vi "Configure Hardware.vi"(8 "error in (no error)":errorcluster, 11 "Hardware Resources in":T2={"VISA resource name"="", "DAQ Type"=0, "Channel 1"={"Acquiring"=FALSE, "Enabled"=FALSE, "Terminal configuration"=32767, "Range"=0, "Coupling"=0}, "Channel 2"={"Acquiring"=FALSE, "Enabled"=FALSE, "Terminal configuration"=0, "Range"=0, "Coupling"=0}, "Timing"={"Sample Time [Time Units]"=0, "Actual Sample Time [s]"=0.0, "Samples per Iteration"=0, "Sample Clock Source"=0, "Time Units"=0, "t0"=timestamp(0 s since 1904-01-01), "Baud rate"=0}, "PS Parameters"={"PS handle"=0, "PS Max_adc"=32767, "PS Enabled Array"=[], "PS Device Info"={"Driver Version"="", "USB Version"="", "Hardware"="", "Variant"="", "Batch and Serial"="", "Cal Date"="", "Kernel Version"="", "Digital HW Version"="", "Analogue HW Version"="", "Firmware 1"="", "Firmware 2"="", "MSO"=FALSE, "Number of Channels"=0}, "Channel 1 Buffer"=refnum, "Channel 2 Buffer"=refnum, "Resolution"=0, "USB Power"=FALSE}, "Trigger"={"Direction"=0, "Threshold [V]"=0.0, "Enabled"=FALSE, "Trigger Source"=0}, "Keithley Parameters"={"Previous End / Current Start"=0, "Quantity"=0}} {"Keithley Parameters"."Quantity" items=["Current", "Voltage"]; "Trigger"."Trigger Source" items=["Channel 1"=0, "Channel 2"=1, "Ext."=4]; "Trigger"."Direction" items=["Falling", "Rising"]; "PS Parameters"."Resolution" items=["8", "12", "14", "15", "16"]; "Timing"."Time Units" items=["Seconds"]; "Timing"."Sample Clock Source" items=["Internal", "External"]; "Channel 2"."Coupling" items=["AC", "DC"]; "Channel 2"."Range" items=["0.01", "0.02", "0.05", "0.1", "0.2", "0.5", "1", "2", "5", "10", "20", "50", "100", "1000"]; "Channel 2"."Terminal configuration" items=["Referenced Single Ended", "Differential"]; "Channel 1"."Coupling" items=["AC", "DC"]; "Channel 1"."Range" items=["0.01", "0.02", "0.05", "0.1", "0.2", "0.5", "1", "2", "5", "10", "20", "50", "100", "1000"]; "Channel 1"."Terminal configuration" items=["Referenced Single Ended", "Differential"]; "DAQ Type" items=["Simulated", "Tektronics DPO2k/3k/4k", "PicoScope 2000a Series", "Keithley DMM7510", "PicoScope 5000a Series", "Arduino"]}) -> (0 "error out":errorcluster, 3 "Hardware Resources out":T2={"VISA resource name"="", "DAQ Type"=0, "Channel 1"={"Acquiring"=FALSE, "Enabled"=FALSE, "Terminal configuration"=32767, "Range"=0, "Coupling"=0}, "Channel 2"={"Acquiring"=FALSE, "Enabled"=FALSE, "Terminal configuration"=0, "Range"=0, "Coupling"=0}, "Timing"={"Sample Time [Time Units]"=0, "Actual Sample Time [s]"=0.0, "Samples per Iteration"=0, "Sample Clock Source"=0, "Time Units"=0, "t0"=timestamp(0 s since 1904-01-01), "Baud rate"=0}, "PS Parameters"={"PS handle"=0, "PS Max_adc"=32767, "PS Enabled Array"=[], "PS Device Info"={"Driver Version"="", "USB Version"="", "Hardware"="", "Variant"="", "Batch and Serial"="", "Cal Date"="", "Kernel Version"="", "Digital HW Version"="", "Analogue HW Version"="", "Firmware 1"="", "Firmware 2"="", "MSO"=FALSE, "Number of Channels"=0}, "Channel 1 Buffer"=refnum, "Channel 2 Buffer"=refnum, "Resolution"=0, "USB Power"=FALSE}, "Trigger"={"Direction"=0, "Threshold [V]"=0.0, "Enabled"=FALSE, "Trigger Source"=0}, "Keithley Parameters"={"Previous End / Current Start"=0, "Quantity"=0}} {"Keithley Parameters"."Quantity" items=["Current", "Voltage"]; "Trigger"."Trigger Source" items=["Channel 1"=0, "Channel 2"=1, "Ext."=4]; "Trigger"."Direction" items=["Falling", "Rising"]; "PS Parameters"."Resolution" items=["8", "12", "14", "15", "16"]; "Timing"."Time Units" items=["Seconds"]; "Timing"."Sample Clock Source" items=["Internal", "External"]; "Channel 2"."Coupling" items=["AC", "DC"]; "Channel 2"."Range" items=["0.01", "0.02", "0.05", "0.1", "0.2", "0.5", "1", "2", "5", "10", "20", "50", "100", "1000"]; "Channel 2"."Terminal configuration" items=["Referenced Single Ended", "Differential"]; "Channel 1"."Coupling" items=["AC", "DC"]; "Channel 1"."Range" items=["0.01", "0.02", "0.05", "0.1", "0.2", "0.5", "1", "2", "5", "10", "20", "50", "100", "1000"]; "Channel 1"."Terminal configuration" items=["Referenced Single Ended", "Differential"]; "DAQ Type" items=["Simulated", "Tektronics DPO2k/3k/4k", "PicoScope 2000a Series", "Keithley DMM7510", "PicoScope 5000a Series", "Arduino"]})   [LabVIEW 2017, in "Acquisition.lvlib"]
doc: "Configure the hardware."
uses:
  Acquisition.lvlib
  Hardware Configuration.ctl
  Signal Type.ctl
  Settings/Terminal Configuration.ctl
  Settings/Range.ctl
  Settings/Coupling.ctl
  Settings/Sampling Clock Source.ctl
  Settings/Time Units.ctl
  Settings/Resolution.ctl
  Settings/Trigger Direction.ctl
  Settings/Trigger Source.ctl
  Settings/Quantity.ctl
  support/DAQ Drivers/Tektronix DPO MSO 2000 4000 Series/Tektronix DPO MSO 2000 4000 Series.lvlib
  Settings/Settings.lvlib
panel:
  out "Range":T1 items=["10 u"=50, "100 u"=51, "1 m"=52, "10 m"=0, "20 m"=1, "50 m"=2, "100 m"=3, "200 m"=4, "500 m"=5, "1"=6, "2"=7, "3"=53, "5"=8, "10"=9, "20"=10, "50"=11, "100"=12, "700"=90, "1000"=13]
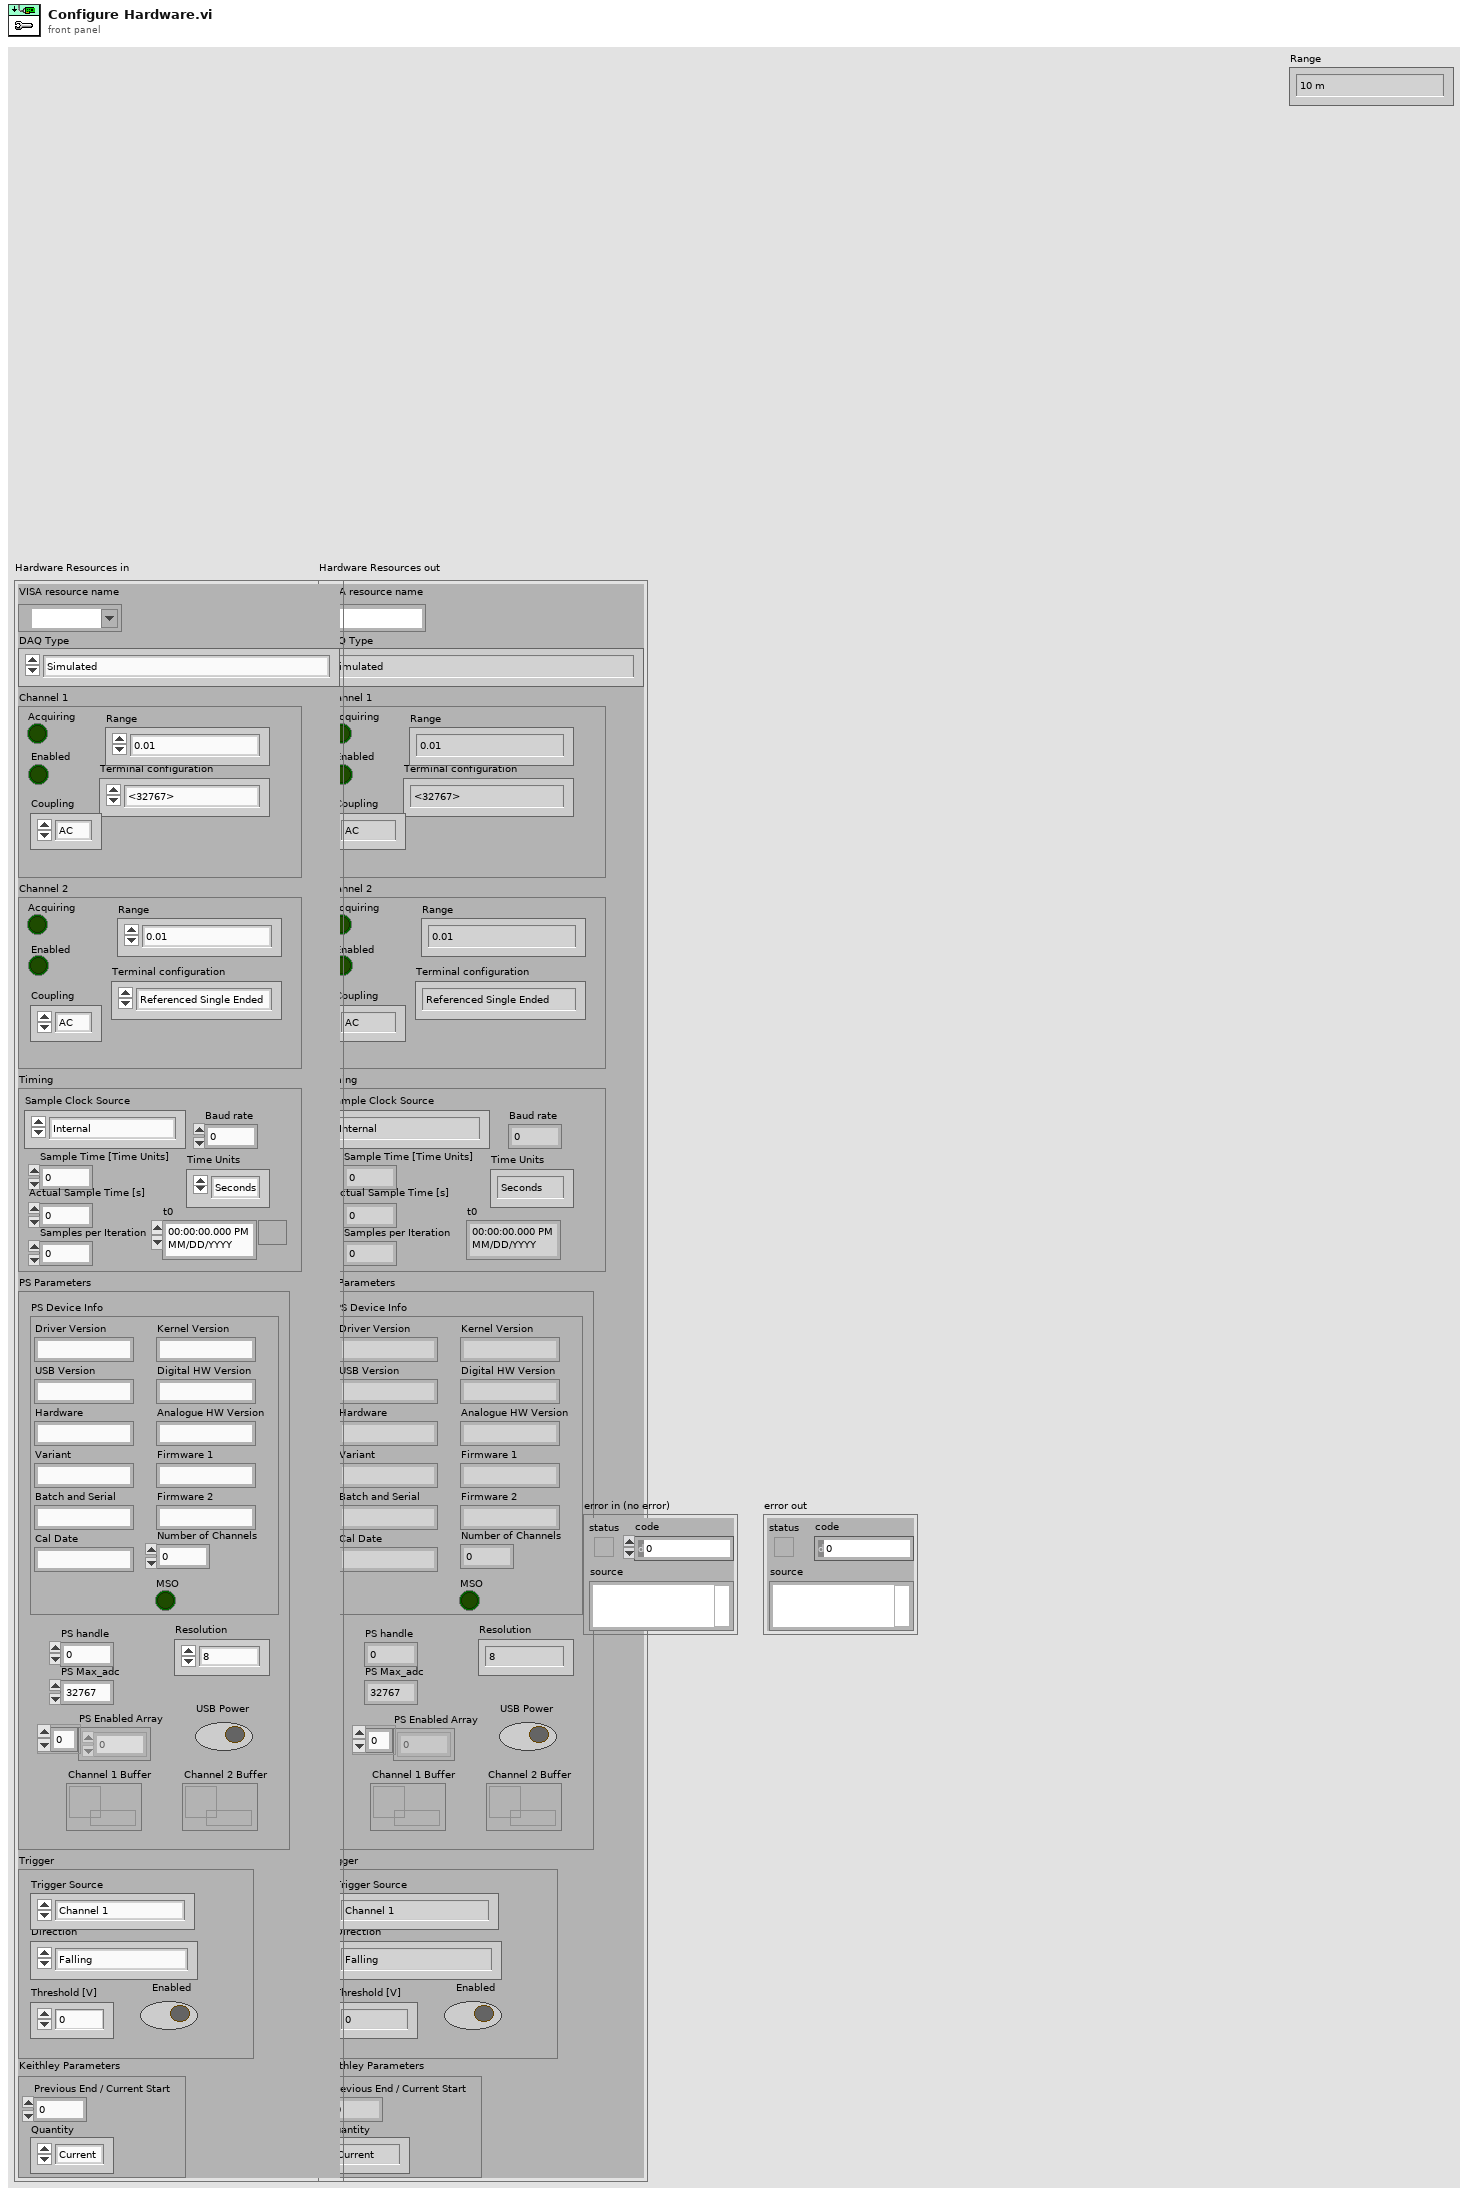
[diagram p1: front panel]
types:
  T1 = typedef "Settings.lvlib/Range.ctl" = u16
  T2 = typedef "Acquisition.lvlib/Hardware Configuration.ctl" = cluster{"VISA resource name":refnum<visa-resource-name>, "DAQ Type":T3, "Channel 1":cluster{"Acquiring":bool, "Enabled":bool, "Terminal configuration":T4, "Range":T1, "Coupling":T5}, "Channel 2":cluster{"Acquiring":bool, "Enabled":bool, "Terminal configuration":T4, "Range":T1, "Coupling":T5}, "Timing":cluster{"Sample Time [Time Units]":u32, "Actual Sample Time [s]":dbl, "Samples per Iteration":u32, "Sample Clock Source":T6, "Time Units":T7, "t0":timestamp, "Baud rate":u32}, "PS Parameters":cluster{"PS handle":i16, "PS Max_adc":i16, "PS Enabled Array":i16[], "PS Device Info":cluster{"Driver Version":string, "USB Version":string, "Hardware":string, "Variant":string, "Batch and Serial":string, "Cal Date":string, "Kernel Version":string, "Digital HW Version":string, "Analogue HW Version":string, "Firmware 1":string, "Firmware 2":string, "MSO":bool, "Number of Channels":i16}, "Channel 1 Buffer":refnum<data-value>, "Channel 2 Buffer":refnum<data-value>, "Resolution":T8, "USB Power":bool}, "Trigger":cluster{"Direction":T9, "Threshold [V]":dbl, "Enabled":bool, "Trigger Source":T10}, "Keithley Parameters":cluster{"Previous End / Current Start":i32, "Quantity":T11}}
  T3 = typedef "Acquisition.lvlib/Signal Type.ctl" = u16
  T4 = typedef "Settings.lvlib/Terminal Configuration.ctl" = u16
  T5 = typedef "Settings.lvlib/Coupling.ctl" = i16
  T6 = typedef "Settings.lvlib/Sampling Clock Source.ctl" = u16
  T7 = typedef "Settings.lvlib/Time Units.ctl" = u32
  T8 = typedef "Settings.lvlib/Resolution.ctl" = i32
  T9 = typedef "Settings.lvlib/Trigger Direction.ctl" = u16
  T10 = typedef "Settings.lvlib/Trigger Source.ctl" = u16
  T11 = typedef "Settings.lvlib/Quantity.ctl" = u16
  T12 = cluster{"Auto Stop":bool, "Desired Sample Interval":u32, "Pre-trigger Samples":u32, "Post-trigger Samples":u32, "Down-Sample Ratio":u32, "Down-Sample Mode":u32, "Overview Buffer Size":i32, "Time Units":u32}
  T13 = cluster{"Trigger Enabled":bool, "Trigger Source":enum16{"Channel A", "Channel B", "Channel C", "Channel D", "Ext."}, "Trigger Threshold (Volts)":dbl, "Trigger Direction":u16, "Trigger Delay (samples)":u32, "Auto Trigger Time (ms)":i16}
  T14 = cluster{"Auto Stop":bool, "Four Channel Device?":bool, "Desired Sample Interval":u32, "Pre-trigger Samples":u32, "Post-trigger Samples":u32, "Down-Sample Ratio":u32, "Down-Sample Mode":i32, "Overview Buffer Size":u32, "Time Units":u32}
  T15 = cluster{"Trigger Enabled":bool, "Trigger Source":enum16{"Channel A", "Channel B", "Channel C", "Channel D", "Ext."}, "Trigger Threshold (16-bit counts)":i16, "Trigger Direction":u16, "Trigger Delay (samples)":u32, "Auto Trigger Time (ms)":i16}
  T16 = cluster{"Acquiring":bool, "Enabled":bool, "Terminal configuration":T4, "Range":T1, "Coupling":T5}
  T17 = cluster{"Sample Time [Time Units]":u32, "Actual Sample Time [s]":dbl, "Samples per Iteration":u32, "Sample Clock Source":T6, "Time Units":T7, "t0":timestamp, "Baud rate":u32}
  T18 = cluster{"PS handle":i16, "PS Max_adc":i16, "PS Enabled Array":i16[], "PS Device Info":cluster{"Driver Version":string, "USB Version":string, "Hardware":string, "Variant":string, "Batch and Serial":string, "Cal Date":string, "Kernel Version":string, "Digital HW Version":string, "Analogue HW Version":string, "Firmware 1":string, "Firmware 2":string, "MSO":bool, "Number of Channels":i16}, "Channel 1 Buffer":refnum<data-value>, "Channel 2 Buffer":refnum<data-value>, "Resolution":T8, "USB Power":bool}
  T19 = cluster{"Direction":T9, "Threshold [V]":dbl, "Enabled":bool, "Trigger Source":T10}
  T20 = cluster{"Previous End / Current Start":i32, "Quantity":T11}
  T21 = cluster{"Enabled":bool, "Coupling":i16, "Range":u16, "Analogue Offset":sgl}
  T22 = cluster{"Driver Version":string, "USB Version":string, "Hardware":string, "Variant":string, "Batch and Serial":string, "Cal Date":string, "Kernel Version":string, "Digital HW Version":string, "Analogue HW Version":string, "Firmware 1":string, "Firmware 2":string, "MSO":bool, "Number of Channels":i16}
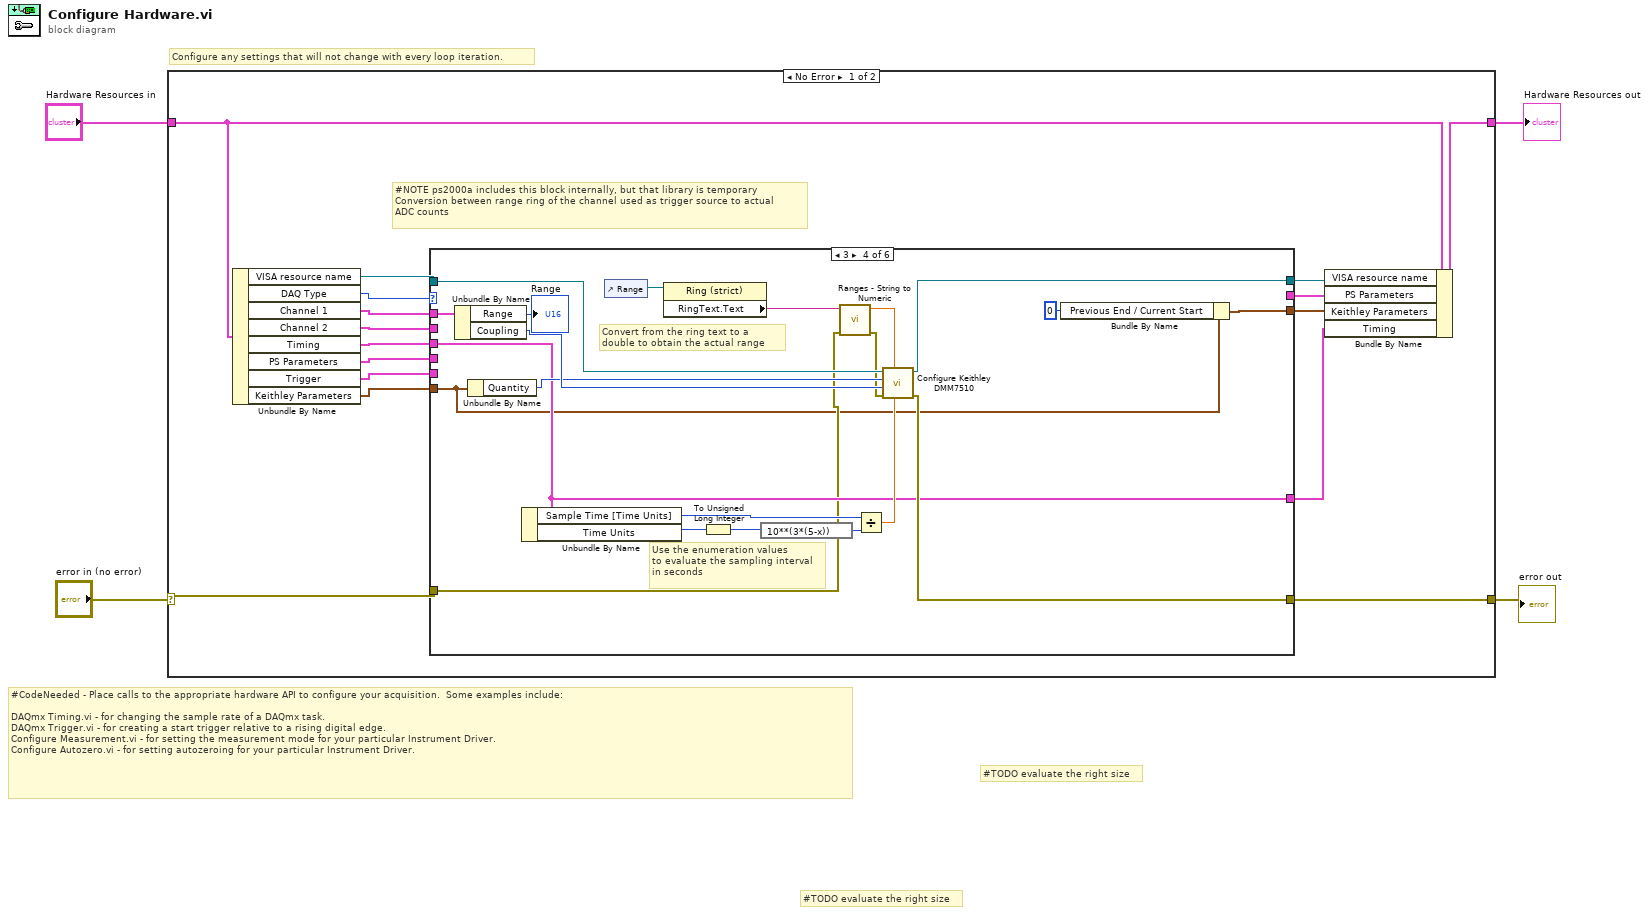
[diagram p0: block diagram]
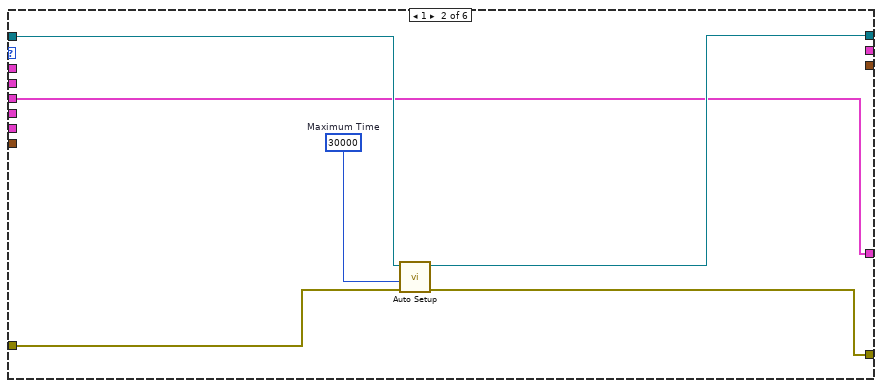
[diagram p3: hidden frame]
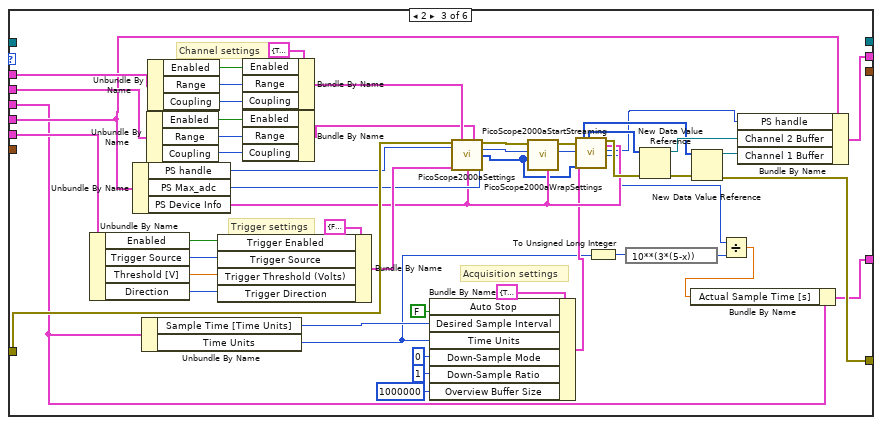
[diagram p4: hidden frame]
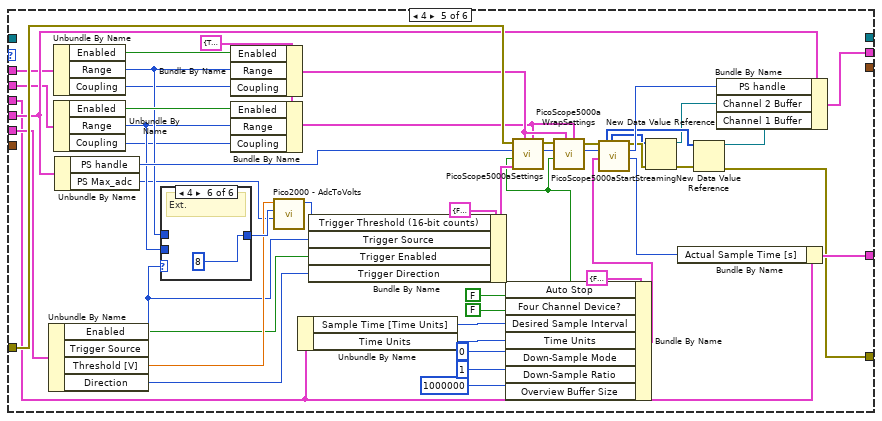
[diagram p5: hidden frame]
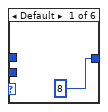
[diagram p6: hidden frame]
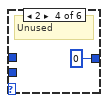
[diagram p9: hidden frame]
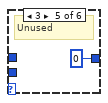
[diagram p10: hidden frame]
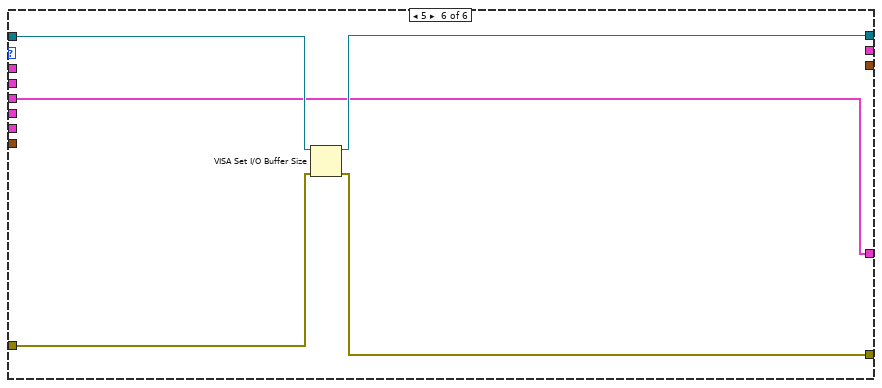
[diagram p11: hidden frame]
diagram:
  # "#TODO evaluate the right size"
  # "#TODO evaluate the right size"
  # "Configure any settings that will not change with every loop iteration."
  # "#CodeNeeded - Place calls to the appropriate hardware API to configure your acquisition.  Some examples include:\n\nDAQmx Timing.vi - for changing the sample rate of a DAQmx task.\nDAQmx Trigger.vi - for creating a start trigger relative to a rising digital edge.\nConfigure Measurement.vi - for setting the measurement mode for your particular Instrument Driver.\nConfigure Autozero.vi - for setting autozeroing for your particular Instrument Driver."
  n1 = case shown="No Error" "error in (no error)" {
    selector: "error in (no error)" -> [w19 w161]
    tunnel: [w18 w161] -> w3
    tunnel: "Hardware Resources in" -> [w16 w162]
    tunnel: [w20 w162] -> w1
    frame No Error {
      # "#NOTE ps2000a includes this block internally, but that library is temporary\nConversion between range ring of the channel used as trigger source to actual\nADC counts"
      n2 = Unbundle By Name(w16) -> ("VISA resource name"=w15:refnum<visa-resource-name>, "DAQ Type"=w14:T3, "Channel 1"=w13:T16, "Channel 2"=w11:T16, "Timing"=w12:T17, "PS Parameters"=w9:T18, "Trigger"=w10:T19, "Keithley Parameters"=w6:T20)
      n3 = case shown="3" w14 {
        tunnel: w19 -> [w22 w28 w77 w84 w149 w157]
        tunnel: [w22 w27 w50 w100 w115 w159] -> w18
        tunnel: [_ w26 _ w99 _ w160] -> w17
        tunnel: w15 -> [_ w24 _ w98 _ w158]
        tunnel: w13 -> [_ _ w73 w95 w137 _]
        tunnel: w12 -> [w21 w23 w41 w88 w121 w156]
        tunnel: w11 -> [_ _ w70 _ w131 _]
        tunnel: w10 -> [_ _ w67 _ w139 _]
        tunnel: w9 -> [_ _ w47 _ w143 _]
        tunnel: [w21 w23 w45 w88 w119 w156] -> w8
        tunnel: [_ _ w46 _ w118 _] -> w7
        tunnel: w6 -> [_ _ _ w81 _ _]
        tunnel: [_ _ _ w82 _ _] -> w5
        frame 0, Default {
        }
        frame 1 {
          w25 = 30000  # Maximum Time
          n4 = call "Auto Setup.vi"("error in (no error)"=w28, "Maximum Time (10000ms)"=w25, "VISA resource name"=w24) -> ("error out"=w27:errorcluster, "VISA resource name out"=w26:refnum<visa-resource-name>)  [unwired: 7 in]
        }
        frame 2 {
          w60 = T21 {"Enabled"=TRUE, "Coupling"=1, "Range"=9, "Analogue Offset"=0.0} ("Channel A Settings")
          # "Trigger settings"
          # "Channel settings"
          # "Acquisition settings"
          n5 = Unbundle By Name(w67) -> ("Enabled"=w66:bool, "Trigger Source"=w65:T10, "Threshold [V]"=w64:dbl, "Direction"=w63:T9)
          n6 = Unbundle By Name(w47) -> ("PS handle"=w62:i16, "PS Max_adc"=w61:i16, "PS Device Info"=w49:T22)
          n7 = Unbundle By Name(w41) -> ("Sample Time [Time Units]"=w36:u32, "Time Units"=w29:T7)
          n8 = Unbundle By Name(w70) -> ("Enabled"=w69:bool, "Range"=w68:T1, "Coupling"=w34:T5)
          n9 = Unbundle By Name(w73) -> ("Enabled"=w72:bool, "Range"=w71:T1, "Coupling"=w35:T5)
          n10 = Bundle By Name(cluster=T13 {"Trigger Enabled"=FALSE, "Trigger Source"=enum."Channel A", "Trigger Threshold (Volts)"=0.0, "Trigger Direction"=0, "Trigger Delay (samples)"=0, "Auto Trigger Time (ms)"=0} ("input cluster"), "Trigger Enabled"=w66, "Trigger Source"=w65, "Trigger Threshold (Volts)"=w64, "Trigger Direction"=w63) -> (w74:T13)
          n11 = Bundle By Name(cluster=w60, "Enabled"=w72, "Range"=w71, "Coupling"=w35) -> (w76:T21)
          n12 = Bundle By Name(cluster=w60, "Enabled"=w69, "Range"=w68, "Coupling"=w34) -> (w75:T21)
          n13 = Bundle By Name(cluster=T12 {"Auto Stop"=TRUE, "Desired Sample Interval"=1, "Pre-trigger Samples"=0, "Post-trigger Samples"=1000000, "Down-Sample Ratio"=1, "Down-Sample Mode"=0, "Overview Buffer Size"=50000, "Time Units"=3} ("Acquisition Settings"), "Auto Stop"=FALSE, "Desired Sample Interval"=w36, "Time Units"=w29, "Down-Sample Mode"=u32 0, "Down-Sample Ratio"=u32 1, "Overview Buffer Size"=1000000) -> (w43:T12)
          n14 = call "PicoScope2000aSettings.vi"("error in"=w77, "Channel A Settings"=w76, "Channel B Settings"=w75, "handle in"=w62, "Trigger Settings"=w74, "Device Info"=w49, "Max_adc"=w61) -> ("error out"=w79:errorcluster, "handle out"=w78:i16, "Enabled Array"=w48:i16[])  [unwired: 6 in]
          n15 = call "PicoScope2000aWrapSettings.vi"("Device Info"=w49, "Enabled array"=w48, "Handle In"=w78, "error in (no error)"=w79) -> ("Handle Out"=w57:i16, "error out"=w58:errorcluster)  [unwired: 6 in]
          n16 = call "PicoScope2000aStartStreaming.vi"("error in"=w58, "handle in"=w57, "Acquisition Settings"=w43, "Enabled Array"=w48, "Device Info"=w49) -> ("Channel A"=w52:i16[], "Channel B"=w53:i16[], "error out"=w51:errorcluster, "handle out"=w37:i16, "Sample Interval"=w31:u32)  [unwired: 10 out]
          n17 = To Unsigned Long Integer(number=w29) -> (unsigned 32bit integer=w32:T7)
          n18 = expression code="10**(3*(5-x))"(w32) -> (w33:T7)
          n19 = New Data Value Reference(data value=w53, error in=w51) -> (data value reference=w54:refnum<data-value>, error out=w56:errorcluster)
          n20 = New Data Value Reference(data value=w52, error in=w56) -> (data value reference=w55:refnum<data-value>, error out=w50:errorcluster)
          n21 = Divide(x=w31, y=w33) -> (x/y=w30:dbl)
          n22 = Bundle By Name(cluster=w41, "Actual Sample Time [s]"=w30) -> (w45:T17)
          n23 = Bundle By Name(cluster=w47, "PS handle"=w37, "Channel 2 Buffer"=w54, "Channel 1 Buffer"=w55) -> (w46:T18)
        }
        frame 3 {
          # "Convert from the ring text to a double to obtain the actual range"
          # "Use the enumeration values\nto evaluate the sampling interval\nin seconds"
          n24 = Unbundle By Name(w95) -> ("Range"=→"Range":T1, "Coupling"=w92:T5)
          n25 = Unbundle By Name(w81) -> ("Quantity"=w91:T11)
          n26 = Unbundle By Name(w88) -> ("Sample Time [Time Units]"=w96:u32, "Time Units"=w90:T7)
          n27 = control-ref of="Range"() -> (w83:refnum<vi>)
          n28 = property class="Ring (strict)"(reference=w83) -> ("RingText.Text"=w87:string)  [unwired: 1 in, 2 out]
          n29 = To Unsigned Long Integer(number=w90) -> (unsigned 32bit integer=w89:T7)
          n30 = expression code="10**(3*(5-x))"(w89) -> (w93:T7)
          n31 = call "Ranges - String to Numeric.vi"("error in"=w84, "String"=w87) -> ("error out"=w85:errorcluster, "Numeric"=w86:dbl)  [unwired: 8 in]
          n32 = Divide(x=w96, y=w93) -> (x/y=w97:dbl)
          n33 = call "Configure Keithley DMM7510.vi"("Sampling interval [s]"=w97, "Manual Range"=w86, "error in (no error)"=w85, "Coupling"=w92, "Quantity"=w91, "VISA resource name"=w98) -> ("error out"=w100:errorcluster, "VISA resource name out"=w99:refnum<visa-resource-name>)  [unwired: 4 in]
          n34 = Bundle By Name(cluster=w81, "Previous End / Current Start"=0) -> (w82:T20)
        }
        frame 4 {
          w134 = T21 {"Enabled"=TRUE, "Coupling"=1, "Range"=6, "Analogue Offset"=0.0} ("Channel A Settings")
          w128 = FALSE ("Four Channel Device?")
          n35 = Unbundle By Name(w139) -> ("Enabled"=w101:bool, "Trigger Source"=w102:T10, "Threshold [V]"=w107:dbl, "Direction"=w138:T9)
          n36 = Unbundle By Name(w137) -> ("Enabled"=w136:bool, "Range"=w109:T1, "Coupling"=w105:T5)
          n37 = Unbundle By Name(w131) -> ("Enabled"=w135:bool, "Range"=w108:T1, "Coupling"=w104:T5)
          n38 = Unbundle By Name(w143) -> ("PS handle"=w148:i16, "PS Max_adc"=w106:i16)
          n39 = case shown="4" w102 {
            tunnel: [u16 8 ("Range") w151 w152 u16 0 ("Range") u16 0 ("Range") u16 8 ("Range")] -> w110
            tunnel: w109 -> [_ w151 _ _ _ _]
            tunnel: w108 -> [_ _ w152 _ _ _]
            frame Default {
            }
            frame 0 {
              # "Channel A"
            }
            frame 1 {
              # "Channel B"
            }
            frame 2 {
              # "Unused"
            }
            frame 3 {
              # "Unused"
            }
            frame 4 {
              # "Ext."
            }
          }
          n40 = Bundle By Name(cluster=w134, "Enabled"=w136, "Range"=w109, "Coupling"=w105) -> (w133:T21)
          n41 = Bundle By Name(cluster=w134, "Enabled"=w135, "Range"=w108, "Coupling"=w104) -> (w132:T21)
          n42 = call "Pico2000 - AdcToVolts.vi"("Max ADC"=w106, "Range Index"=w110, "Data (Volts)"=w107) -> ("Data (ADC counts)"=w103:i16)  [unwired: 8 in]
          n43 = Unbundle By Name(w121) -> ("Sample Time [Time Units]"=w127:u32, "Time Units"=w123:T7)
          n44 = Bundle By Name(cluster=T15 {"Trigger Enabled"=FALSE, "Trigger Source"=enum."Channel A", "Trigger Threshold (16-bit counts)"=0, "Trigger Direction"=2, "Trigger Delay (samples)"=0, "Auto Trigger Time (ms)"=1000} ("Trigger Settings"), "Trigger Threshold (16-bit counts)"=w103, "Trigger Source"=w102, "Trigger Enabled"=w101, "Trigger Direction"=w138) -> (w140:T15)
          n45 = Bundle By Name(cluster=T14 {"Auto Stop"=FALSE, "Four Channel Device?"=FALSE, "Desired Sample Interval"=1000, "Pre-trigger Samples"=0, "Post-trigger Samples"=1000, "Down-Sample Ratio"=1, "Down-Sample Mode"=0, "Overview Buffer Size"=15000, "Time Units"=0} ("Acquisition Settings"), "Auto Stop"=FALSE, "Four Channel Device?"=w128, "Desired Sample Interval"=w127, "Time Units"=w123, "Down-Sample Mode"=0, "Down-Sample Ratio"=u32 1 ("Post-trigger Samples"), "Overview Buffer Size"=u32 1000000) -> (w122:T14)
          n46 = call "PicoScope5000aSettings.vi"("Channel B Settings"=w132, "Channel A Settings"=w133, "Trigger Settings"=w140, "Four Channel Device?"=w128, "handle in"=w148, "error in"=w149) -> ("handle out"=w146:i16, "error out"=w147:errorcluster)  [unwired: 4 in]
          n47 = call "PicoScope5000aWrapSettings.vi"("Channel B Settings"=w132, "Channel A Settings"=w133, "Four Channel Device?"=w128, "Handle In"=w146, "error in (no error)"=w147) -> ("Handle Out"=w144:i16, "error out"=w145:errorcluster)  [unwired: 5 in]
          n48 = call "PicoScope5000aStartStreaming.vi"("error in"=w145, "handle in"=w144, "Acquisition Settings"=w122) -> ("Channel A"=w113:i16[], "Channel B"=w114:i16[], "error out"=w117:errorcluster, "handle out"=w142:i16, "Sample Interval"=w120:u32)  [unwired: 6 in, 6 out]
          n49 = New Data Value Reference(data value=w114, error in=w117) -> (data value reference=w111:refnum<data-value>, error out=w116:errorcluster)
          n50 = Bundle By Name(cluster=w121, "Actual Sample Time [s]"=w120) -> (w119:T17)
          n51 = New Data Value Reference(data value=w113, error in=w116) -> (data value reference=w112:refnum<data-value>, error out=w115:errorcluster)
          n52 = Bundle By Name(cluster=w143, "PS handle"=w142, "Channel 2 Buffer"=w111, "Channel 1 Buffer"=w112) -> (w118:T18)
        }
        frame 5 {
          n53 = VISA Set I/O Buffer Size(VISA resource name=w158, error in (no error)=w157) -> (VISA resource name out=w160:refnum<visa-resource-name>, error out=w159:errorcluster)  [unwired: 2 in]
        }
      }
      n54 = Bundle By Name(cluster=w16, "VISA resource name"=w17, "PS Parameters"=w7, "Keithley Parameters"=w5, "Timing"=w8) -> (w20:T2)
    }
    frame Error {
    }
  }
  "Hardware Resources out" <- w1
  "error out" <- w3
